vi "PPL_Teleop_System_Execute.vi"(11 "Teleop Elapsed Seconds":dbl) -> ()   [LabVIEW 2019]
uses:
  <vilib>/Rock Robotics/Network Tables/NT Write Numeric Array.vi
  <vilib>/Rock Robotics/Network Tables/NT Write Boolean Array.vi
  <vilib>/Rock Robotics/WPI/ThirdParty/JAS_Junk/TrajLib/Trajectory_Library.lvlib
  <vilib>/Rock Robotics/WPI/Joystick/XBox Buttons Indexer.ctl
  <vilib>/Rock Robotics/WPI/Joystick/XBox Axes Indexer.ctl
  <vilib>/Rock Robotics/WPI/Joystick/WPI_JoystickArcadeMapping.vi
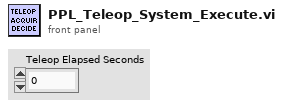
[diagram p1: front panel]
types:
  T1 = typedef "XBox Buttons Indexer.ctl" = enum16{"A", "B", "X", "Y", "Left Bumper", "Right Bumper", "Back", "Start", "Left Joystick", "Right Joystick"}
  T2 = typedef "XBox Axes Indexer.ctl" = enum16{"Left X", "Left Y", "Left Trigger", "Right Trigger", "Right X", "Right Y"}
  T3 = typedef "WPI_JoystickDevRef.ctl" = cluster{"Device":T4}
  T4 = typedef "WPI_JoystickDeviceEnum.ctl" = enum16{"USB 0", "USB 1", "USB 2", "USB 3", "USB 4", "USB 5"}
  T5 = typedef "Trajectory_Library.lvlib/POSE2D.ctl" = cluster{"TRANSLATION":T6, "ROTATION":T7}
  T6 = typedef "Trajectory_Library.lvlib/TRANSLATION2D.ctl" = cluster{"X":dbl, "Y":dbl}
  T7 = typedef "Trajectory_Library.lvlib/ROTATION2D.ctl" = cluster{"VALUE":dbl, "COS":dbl, "SIN":dbl}
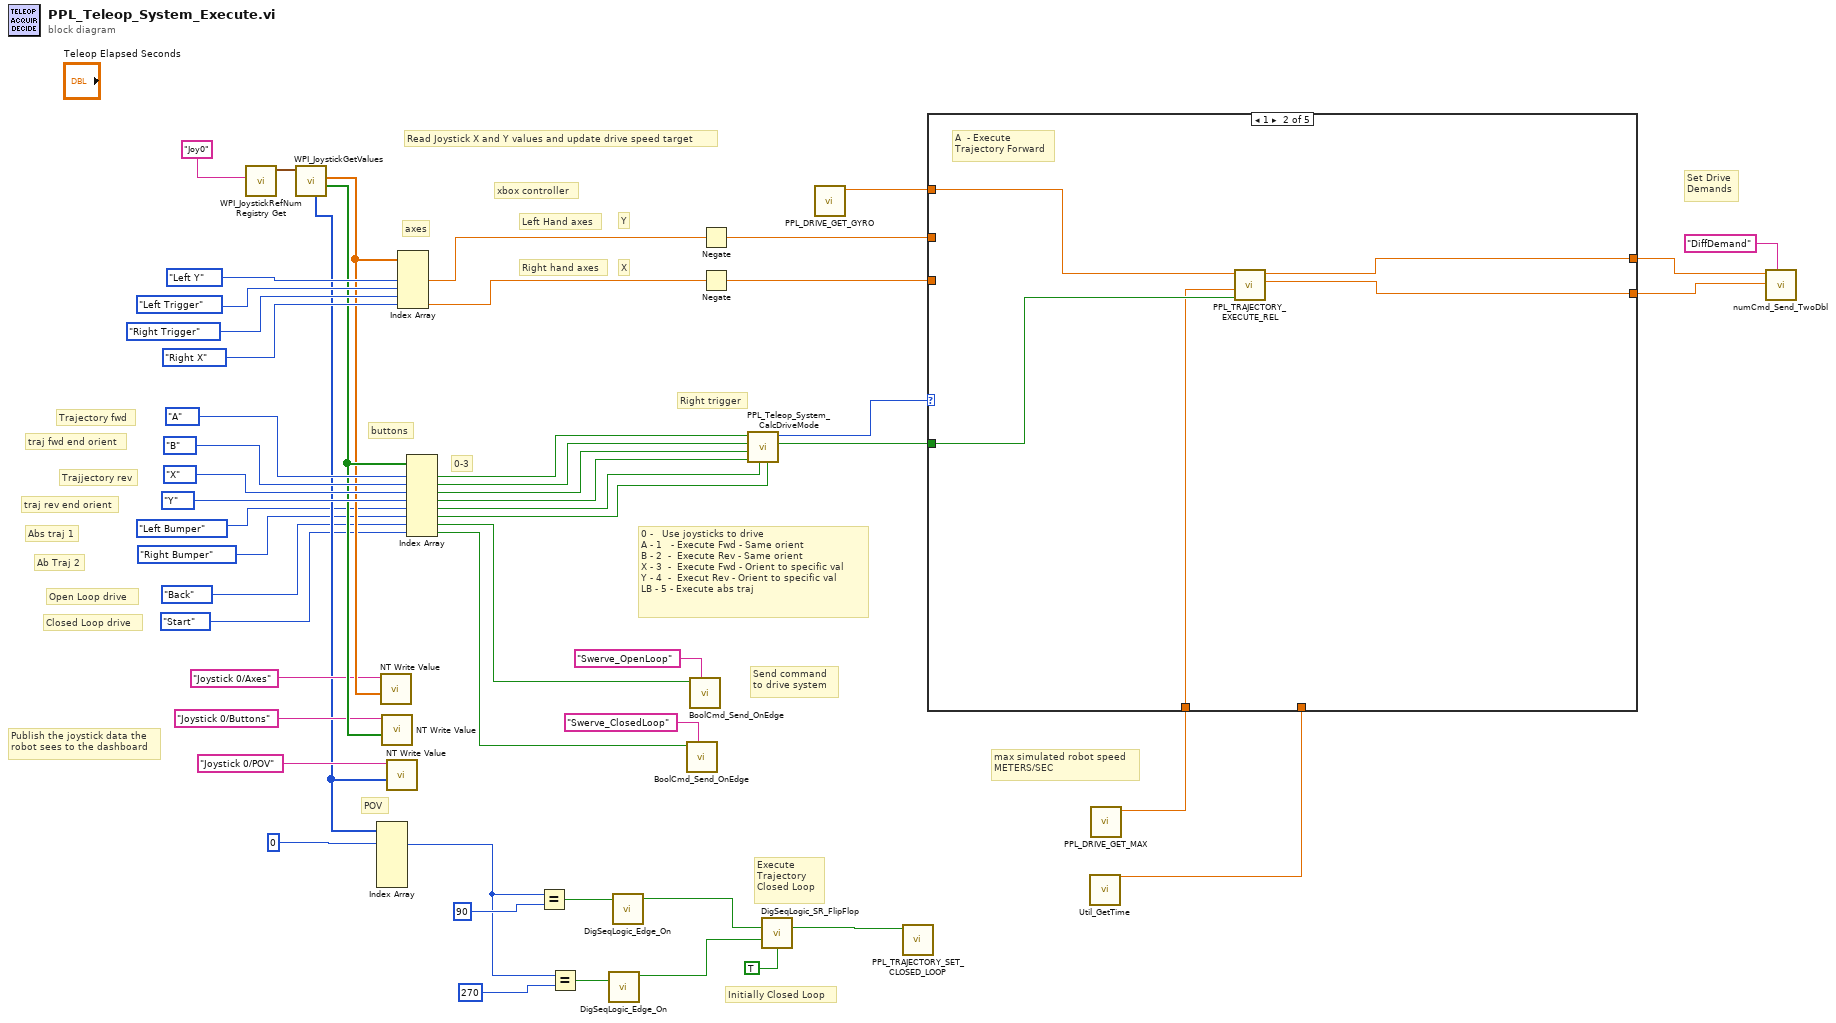
[diagram p0: block diagram]
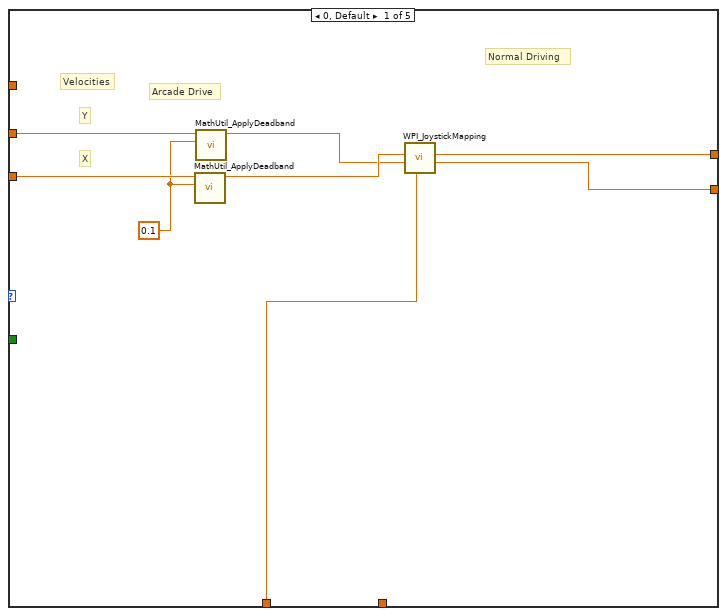
[diagram p2: hidden frame]
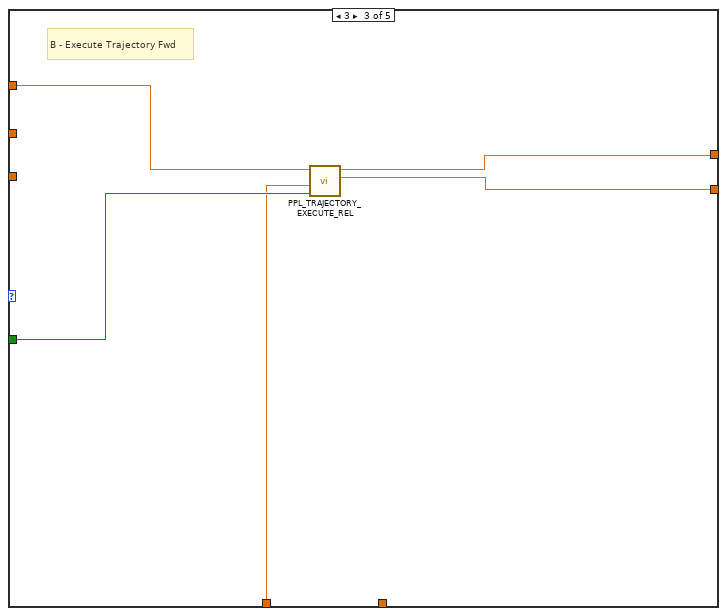
[diagram p3: hidden frame]
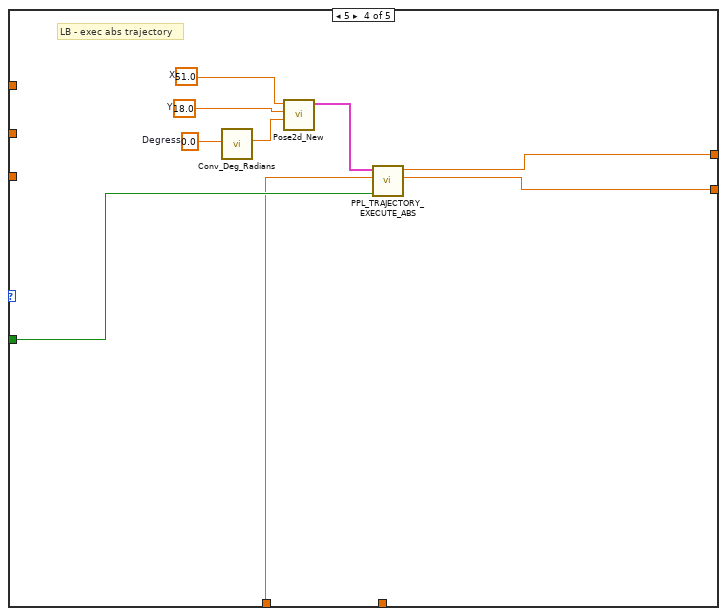
[diagram p4: hidden frame]
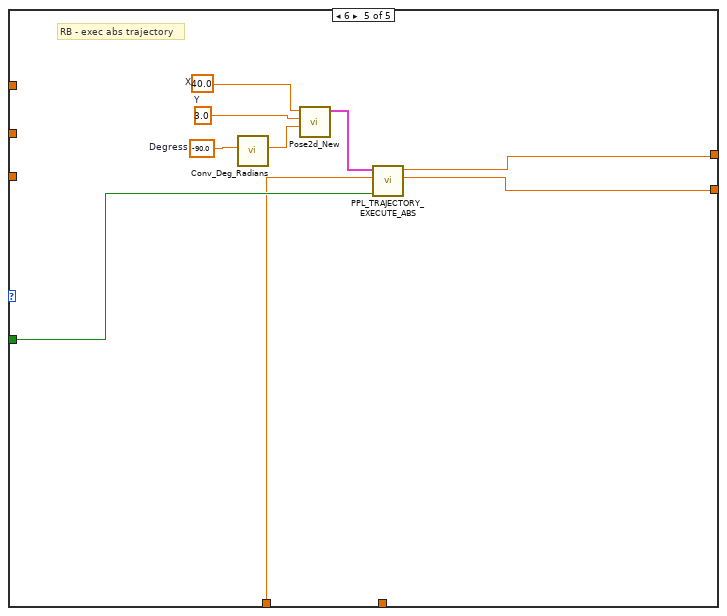
[diagram p5: hidden frame]
diagram:
  # "Send command\nto drive system"
  # "Ab Traj 2"
  # "Abs traj 1"
  # "POV"
  # "traj rev end orient"
  # "traj fwd end orient"
  # "Trajjectory rev"
  # "Closed Loop drive"
  # "Open Loop drive"
  # "Trajectory fwd"
  # "0 -   Use joysticks to drive\nA - 1   - Execute Fwd - Same orient\nB - 2  -  Execute Rev - Same orient\nX - 3  -  Execute Fwd - Orient to specific val\nY - 4  -  Execut Rev - Orient to specific val\nLB - 5 - Execute abs traj"
  # "Execute\nTrajectory\nClosed Loop"
  # "Set Drive\nDemands"
  # "Initially Closed Loop"
  # "0-3"
  # "xbox controller"
  # "Right trigger"
  # "Left Hand axes"
  # "Right hand axes"
  # "X"
  # "Y"
  # "buttons"
  # "axes"
  # "max simulated robot speed\nMETERS/SEC"
  # "Publish the joystick data the\nrobot sees to the dashboard"
  # "Read Joystick X and Y values and update drive speed target"
  n1 = call <vilib>:"WPI_JoystickRefNum Registry Get.vi"("refnum name"="Joy0") -> ("JoystickDevRef"=w27:T3)  [unwired: 1 in, 9 out]
  n2 = call <vilib>:"WPI_JoystickGetValues.vi"("JoystickDevRef"=w27) -> ("Buttons"=w31:bool[], "Axes"=w30:dbl[], "POVs"=w21:i16[])  [unwired: 6 in, 2 out]
  n3 = Index Array(array=w21, index #1=0 ("index")) -> (element #1=w17:i16)  [unwired: 5 in, 5 out]
  n4 = call-poly <vilib>:"NT Write Value.vi"("Numeric Array"=w30, "Name"="Joystick 0/Axes") -> ()  [unwired: 9 in, 1 out]
  n5 = call-poly <vilib>:"NT Write Value.vi"("Boolean Array"=w31, "Name"="Joystick 0/Buttons") -> ()  [unwired: 9 in, 1 out]
  n6 = call-poly <vilib>:"NT Write Value.vi"("Numeric Array"=w21, "Name"="Joystick 0/POV") -> ()  [unwired: 9 in, 1 out]
  n7 = Index Array(array=w30, index #2=XBox_Axes_Indexer."Left Y" ("XBox Axes"), index #3=XBox_Axes_Indexer."Left Trigger" ("XBox Axes"), index #4=XBox_Axes_Indexer."Right Trigger" ("XBox Axes"), index #5=XBox_Axes_Indexer."Right X" ("XBox Axes")) -> (element #2=w38:dbl, element #5=w39:dbl)  [unwired: 1 in, 3 out]
  n8 = Index Array(array=w31, index #1=XBox_Buttons_Indexer."A" ("XBox Buttons"), index #2=XBox_Buttons_Indexer."B" ("XBox Buttons"), index #3=XBox_Buttons_Indexer."X" ("XBox Buttons"), index #4=XBox_Buttons_Indexer."Y" ("XBox Buttons"), index #5=XBox_Buttons_Indexer."Left Bumper" ("XBox Buttons"), index #6=XBox_Buttons_Indexer."Right Bumper" ("XBox Buttons"), index #7=XBox_Buttons_Indexer."Back" ("XBox Buttons"), index #8=XBox_Buttons_Indexer."Start" ("XBox Buttons")) -> (element #1=w32:bool, element #2=w40:bool, element #3=w41:bool, element #4=w48:bool, element #5=w8:bool, element #6=w7:bool, element #7=w4:bool, element #8=w3:bool)
  n9 = Equal?(x=w17, y=i16 90) -> (x = y?=w16:bool)
  n10 = Equal?(x=w17, y=i16 270) -> (x = y?=w15:bool)
  n11 = call <vilib>:"DigSeqLogic_Edge_On.vi"("Input"=w15) -> ("On Edge"=w13:bool)  [unwired: 10 in]
  n12 = call <vilib>:"DigSeqLogic_Edge_On.vi"("Input"=w16) -> ("On Edge"=w14:bool)  [unwired: 10 in]
  n13 = call <vilib>:"BoolCmd_Send_OnEdge.vi"("Command Name"="Swerve_ClosedLoop", "Value"=w3) -> ()  [unwired: 9 in, 1 out]
  n14 = call <vilib>:"BoolCmd_Send_OnEdge.vi"("Command Name"="Swerve_OpenLoop", "Value"=w4) -> ()  [unwired: 9 in, 1 out]
  n15 = Negate(x=w38) -> (-x=w36:dbl)
  n16 = Negate(x=w39) -> (-x=w37:dbl)
  n17 = call "PPL_Teleop_System_CalcDriveMode.vi"("Abs Traj 2"=w7, "Abs Traj 1"=w8, "Traj Rev Follow Orient"=w48, "Traj Rev Same Orient"=w41, "Traj Fwd Follow Orient"=w40, "Traj Fwd Same Orient"=w32) -> ("Dirve Mode Changed"=w34:bool, "Drive Mode"=w33:i32)  [unwired: 4 in]
  n18 = call <vilib>:"DigSeqLogic_SR_FlipFlop.vi"("Set"=w14, "Reset"=w13, "Initial Value"=TRUE) -> ("Output"=w43:bool)  [unwired: 11 in, 1 out]
  n19 = call "PPL_DRIVE_GET_GYRO.vi"() -> ("Gyro Heading Radians"=w24:dbl)  [unwired: 11 in]
  n20 = call "PPL_TRAJECTORY_SET_CLOSED_LOOP.vi"("AUTO_CLOSED_LOOP"=w43) -> ()  [unwired: 11 in]
  n21 = call <vilib>:"Util_GetTime.vi"() -> ("FPGA_Time_Seconds"=w25:dbl)  [unwired: 9 in, 2 out]
  n22 = call "PPL_DRIVE_GET_MAX.vi"() -> ("Max Wheel Vel (Meter/Sec)"=w35:dbl)  [unwired: 10 in, 1 out]
  n23 = case shown="1" w33 {
    tunnel: w37 -> [w59 _ _ _ _]
    tunnel: w35 -> [w57 w61 w66 w71 w82]
    tunnel: w34 -> [_ w65 w70 w79 w88]
    tunnel: w36 -> [w60 _ _ _ _]
    tunnel: w24 -> [_ w64 w69 _ _]
    tunnel: w25 -> [_ _ _ _ _]
    tunnel: [w56 w63 w68 w73 w81] -> w2
    tunnel: [w55 w62 w67 w72 w80] -> w1
    frame 0, Default {
      w58 = 0.1 ("Deadband")
      # "Normal Driving"
      # "Velocities"
      # "X"
      # "Y"
      # "Arcade Drive"
      n24 = call <vilib>:"MathUtil_ApplyDeadband.vi"("Deadband"=w58, "Value"=w59) -> ("Result"=w54:dbl)  [unwired: 9 in]
      n25 = call <vilib>:"MathUtil_ApplyDeadband.vi"("Deadband"=w58, "Value"=w60) -> ("Result"=w53:dbl)  [unwired: 9 in]
      n26 = call-poly <vilib>:"WPI_JoystickMapping.vi"("Max Output"=w57, "Y axis value"=w53, "X axis value"=w54) -> ("Right Motor Value"=w55:dbl, "Left Motor Value"=w56:dbl)  [unwired: 7 in]
    }
    frame 1 {
      # "A  - Execute\nTrajectory Forward"
      n27 = call "PPL_TRAJECTORY_EXECUTE_REL.vi"("Init"=w65, "Max Wheel Speed M/S"=w61, "Gyro Heading\nRAD"=w64) -> ("Right Speed Dmd M/S"=w62:dbl, "Left Speed Dmd M/S"=w63:dbl)  [unwired: 5 in, 2 out]
    }
    frame 3 {
      # "B - Execute Trajectory Fwd"
      n28 = call "PPL_TRAJECTORY_EXECUTE_REL.vi"("Init"=w70, "Max Wheel Speed M/S"=w66, "Gyro Heading\nRAD"=w69) -> ("Right Speed Dmd M/S"=w67:dbl, "Left Speed Dmd M/S"=w68:dbl)  [unwired: 5 in, 2 out]
    }
    frame 5 {
      w75 = 51.0  # X
      w76 = 18.0  # Y
      w77 = 0.0  # Degress
      # "LB - exec abs trajectory"
      n29 = call <vilib>:"Conv_Deg_Radians.vi"("Degress"=w77) -> ("Radians"=w78:dbl)  [unwired: 10 in]
      n30 = call <vilib>:"Pose2d_New.vi"("Heading"=w78, "Y"=w76, "X"=w75) -> ("out POSe"=w74:T5)  [unwired: 8 in]
      n31 = call "PPL_TRAJECTORY_EXECUTE_ABS.vi"("Init"=w79, "Max Wheel Speed M/S"=w71, "End Pose ENG"=w74) -> ("Right Speed Dmd M/S"=w72:dbl, "Left Speed Dmd M/S"=w73:dbl)  [unwired: 6 in, 1 out]
    }
    frame 6 {
      w84 = 40.0  # X
      w85 = 3.0  # Y
      w86 = -90.0  # Degress
      # "RB - exec abs trajectory"
      n32 = call <vilib>:"Conv_Deg_Radians.vi"("Degress"=w86) -> ("Radians"=w87:dbl)  [unwired: 10 in]
      n33 = call <vilib>:"Pose2d_New.vi"("Heading"=w87, "Y"=w85, "X"=w84) -> ("out POSe"=w83:T5)  [unwired: 8 in]
      n34 = call "PPL_TRAJECTORY_EXECUTE_ABS.vi"("Init"=w88, "Max Wheel Speed M/S"=w82, "End Pose ENG"=w83) -> ("Right Speed Dmd M/S"=w80:dbl, "Left Speed Dmd M/S"=w81:dbl)  [unwired: 6 in, 1 out]
    }
  }
  n35 = call <vilib>:"numCmd_Send_TwoDbl.vi"("Command Name"="DiffDemand", "Value 2"=w1, "Value 1"=w2) -> ()  [unwired: 8 in, 1 out]
